vi "Automagic Ultrasonic Shooting.vi"   [LabVIEW 2017]
uses:
  <vilib>/Rock Robotics/WPI/Ultrasonic/WPI_UltrasonicRangeUnits.ctl
  <vilib>/Rock Robotics/WPI/Ultrasonic/WPI_SonarSRF04DigitalRefNum Registry Get.vi
  <vilib>/Rock Robotics/WPI/Ultrasonic/WPI_SonarSRF04DigitalGetRange.vi
  <vilib>/Rock Robotics/WPI/Utilities/WPI_GetSetVariantRefNum.vi
types:
  T1 = typedef "WPI_UltrasonicRangeUnits.ctl" = enum16{"inches", "mm"}
  T2 = typedef "WPI_UltrasonicDeviceRef.ctl" = cluster{"DevStatus":errorcluster, "Ping Channel":T3, "Echo Channel":T3, "CntIndex":T4}
  T3 = typedef "FPGA_DIOChannel.ctl" = enum8{"DIO 0", "DIO 1", "DIO 2", "DIO 3", "DIO 4", "DIO 5", "DIO 6", "DIO 7", "DIO 8", "DIO 9", "DIO MXP 0", "DIO MXP 1", "DIO MXP 2", "DIO MXP 3", "DIO MXP 4", "DIO MXP 5", "DIO MXP 6", "DIO MXP 7", "DIO MXP 8", "DIO MXP 9", "DIO MXP 10", "DIO MXP 11", "DIO MXP 12", "DIO MXP 13", "DIO MXP 14", "DIO MXP 15", "SPI Port CS1", "SPI Port CS2", "SPI Port CS3", "SPI Port MISO", "SPI Port MOSI", "Invalid"}
  T4 = typedef "FPGA_CounterCtrSystemIndex.ctl" = enum8{"Ctr 0", "Ctr 1", "Ctr 2", "Ctr 3", "Ctr 4", "Ctr 5", "Ctr 6", "Ctr 7", "Invalid"}
  T5 = typedef "WPI_RobotDriveDevRef.ctl" = cluster{"DevStatus":errorcluster, "Motors[]":T6[], "Square Inputs":bool, "Max Output":dbl}
  T6 = typedef "WPI_MotorControlDeviceRef.ctl" = cluster{"DeviceStatus":errorcluster, "Type":T7, "PWM":cluster{"PWM Channel":T8, "DeadBand":T9}, "CAN":cluster{"Device Number":u8, "SetOutput VI Ref":variant, "GetOutput VI Ref":variant, "Enable VI Ref":variant, "Disable VI Ref":variant, "Data":variant}, "Invert":bool, "DIO PWM":cluster{"PWM \"Enable\" Channel":T8, "DIOChannel":T3, "PWM Rate":dbl}}
  T7 = typedef "WPI_MotorControlType.ctl" = enum16{"PWM", "CAN", "DIO PWM"}
  T8 = typedef "FPGA_DIOPWMChannel.ctl" = enum8{"PWM 0", "PWM 1", "PWM 2", "PWM 3", "PWM 4", "PWM 5", "PWM 6", "PWM 7", "PWM 8", "PWM 9", "PWM MXP 0", "PWM MXP 1", "PWM MXP 2", "PWM MXP 3", "PWM MXP 4", "PWM MXP 5", "PWM MXP 6", "PWM MXP 7", "PWM MXP 8", "PWM MXP 9", "Invalid"}
  T9 = typedef "WPI_PWMDeadband.ctl" = cluster{"Name":string, "maxPositivePwm":i32, "minPositivePwm":i32, "centerPwm":i32, "maxNegativePwm":i32, "minNegativePwm":i32, "angularRange":u16}
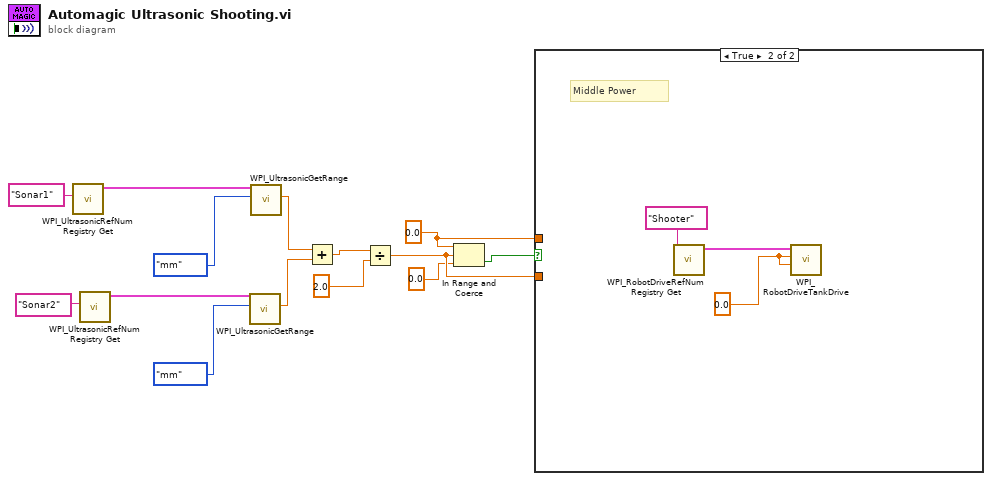
[diagram p0: block diagram]
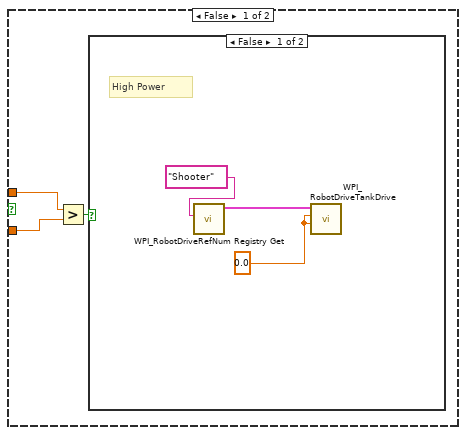
[diagram p2: hidden frame]
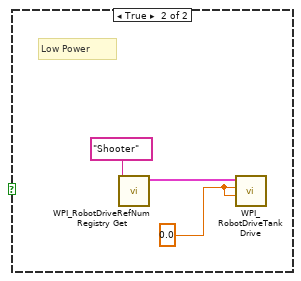
[diagram p3: hidden frame]
diagram:
  w13 = 0.0 ("upper limit")
  n1 = call-poly <vilib>:"WPI_UltrasonicRefNum Registry Get.vi"("refnum name"="Sonar1") -> ("SonarSRF04DevRef"=w2:T2)  [unwired: 9 in, 1 out]
  n2 = call-poly <vilib>:"WPI_UltrasonicRefNum Registry Get.vi"("refnum name"="Sonar2") -> ("SonarSRF04DevRef"=w6:T2)  [unwired: 9 in, 1 out]
  n3 = call-poly <vilib>:"WPI_UltrasonicGetRange.vi"("Range Units"=WPI_UltrasonicRangeUnits."mm", "UltrasonicDevRef"=w6) -> ("Distance"=w8:dbl)  [unwired: 7 in, 2 out]
  n4 = call-poly <vilib>:"WPI_UltrasonicGetRange.vi"("Range Units"=WPI_UltrasonicRangeUnits."mm", "UltrasonicDevRef"=w2) -> ("Distance"=w7:dbl)  [unwired: 7 in, 2 out]
  n5 = Add(x=w7, y=w8) -> (x+y=w9:dbl)
  n6 = Divide(x=w9, y=2.0) -> (x/y=w14:dbl)
  n7 = In Range and Coerce(upper limit=w13, x=w14, lower limit=0.0) -> (In Range?=w12:bool)  [unwired: 1 out]
  n8 = case shown="True" w12 {
    tunnel: w13 -> [w16 _]
    tunnel: w14 -> [w15 _]
    frame False {
      n9 = Greater?(x=w16, y=w15) -> (0:w17:bool)
      n10 = case shown="False" w17 {
        frame False {
          w18 = 0.0 ("Left axis value")
          # "High Power"
          n11 = call <vilib>:"WPI_RobotDriveRefNum Registry Get.vi"("refnum name"="Shooter") -> ("RobotDriveDevRef"=w20:T5)  [unwired: 9 in, 1 out]
          n12 = call <vilib>:"WPI_RobotDriveTankDrive.vi"("Right axis value"=w18, "Left axis value"=w18, "RobotDriveDevRef"=w20) -> ()  [unwired: 6 in, 3 out]
        }
        frame True {
          w21 = 0.0 ("Left axis value")
          # "Low Power"
          n13 = call <vilib>:"WPI_RobotDriveRefNum Registry Get.vi"("refnum name"="Shooter") -> ("RobotDriveDevRef"=w23:T5)  [unwired: 9 in, 1 out]
          n14 = call <vilib>:"WPI_RobotDriveTankDrive.vi"("Right axis value"=w21, "Left axis value"=w21, "RobotDriveDevRef"=w23) -> ()  [unwired: 6 in, 3 out]
        }
      }
    }
    frame True {
      w24 = 0.0 ("Left axis value")
      # "Middle Power"
      n15 = call <vilib>:"WPI_RobotDriveRefNum Registry Get.vi"("refnum name"="Shooter") -> ("RobotDriveDevRef"=w26:T5)  [unwired: 9 in, 1 out]
      n16 = call <vilib>:"WPI_RobotDriveTankDrive.vi"("Right axis value"=w24, "Left axis value"=w24, "RobotDriveDevRef"=w26) -> ()  [unwired: 6 in, 3 out]
    }
  }
